vi "Sandbox.vi"() -> ()   [LabVIEW 2019, in "Logger.lvclass"]
uses:
  Logger.lvclass
  ObjData.ctl
  ObjType.ctl
  SignalData.ctl
  EventData.ctl
  TypeDef/AlarmType.ctl
  Database_Postgress_class/Database_Postgress.lvclass
  D:/GIT H4000/H4000/src/DatabaseInterface_class/DatabaseInterface.lvclass
  Database_Postgress_class/Connection Info.ctl
  Logger.lvclass/Logger.ctl
  DatabaseInterface_class/DatabaseInterface.lvclass
panel:
  in  "Events 2":T1[](array[typedef])=[{"obj_tag"="o_tag_1", "event_tag"="o_tag_1_di", "Description"="dsfsadf", "ALARM TYPE"=enum."Alarm", "Value DBL"=234.0, "Value INT"=23423, "Value STR"="xfddf", "Time Stamp"=timestamp(3831350232.4442434 s since 1904-01-01)}]
  in  "sig":T3[](array[typedef])=[{"Value"=1.0, "SignalTag"="s_tag_1", "ObjTag"="o_tag_1", "Desc"="dfs", "Time Stamp"=timestamp(3831177088.422016 s since 1904-01-01)}, {"Value"=2.0, "SignalTag"="s_tag_1", "ObjTag"="o_tag_1", "Desc"="dfas", "Time Stamp"=timestamp(3831263490.641324 s since 1904-01-01)}, {"Value"=3.0, "SignalTag"="s_tag_2", "ObjTag"="o_tag_1", "Desc"="dfsd", "Time Stamp"=timestamp(3830140293.1623626 s since 1904-01-01)}]
  in  "Array":T4[](array[typedef])=[{"object_tag"="o_tag", "parent_tag"="p_tag", "object_type"=enum."Device", "description"="Тестовый обект"}]
  out "error out":errorcluster
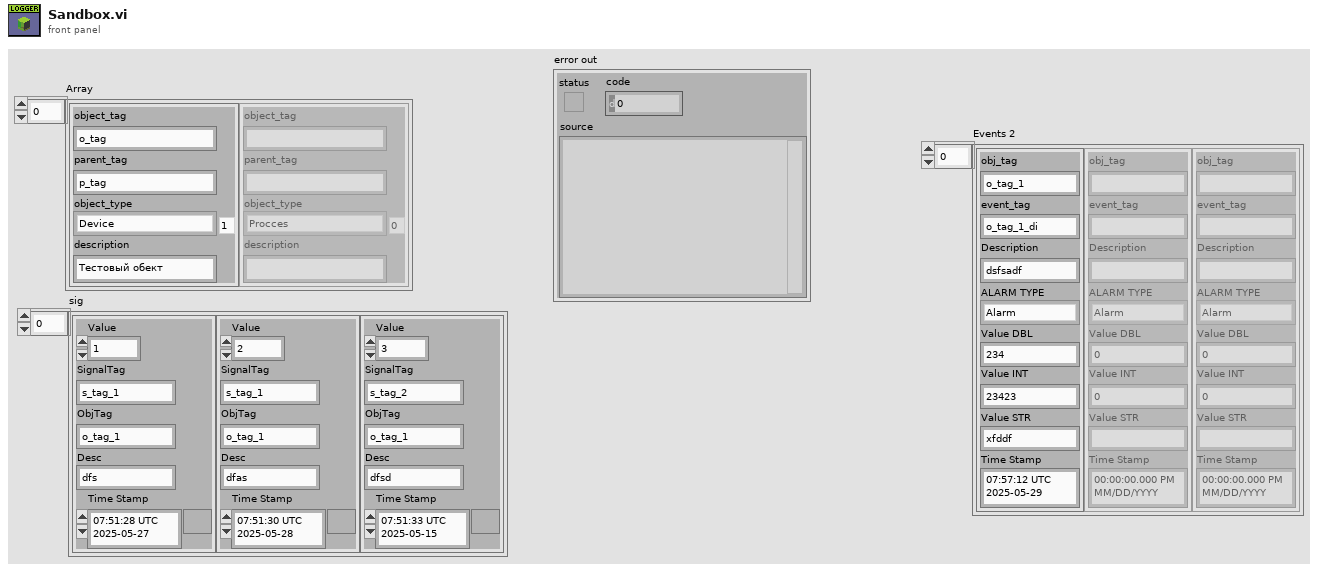
[diagram p1: front panel]
types:
  T1 = typedef "Logger.lvclass/EventData.ctl" = cluster{"obj_tag":string, "event_tag":string, "Description":string, "ALARM TYPE":T2, "Value DBL":dbl, "Value INT":i32, "Value STR":string, "Time Stamp":timestamp}
  T2 = typedef "AlarmType.ctl" = enum16{"Normal", "Warning", "Alarm"}
  T3 = typedef "Logger.lvclass/SignalData.ctl" = cluster{"Value":dbl, "SignalTag":string, "ObjTag":string, "Desc":string, "Time Stamp":timestamp}
  T4 = typedef "Logger.lvclass/ObjData.ctl" = cluster{"object_tag":string, "parent_tag":string, "object_type":T5, "description":string}
  T5 = typedef "Logger.lvclass/ObjType.ctl" = enum16{"Procces", "Device", "Signal", "DI", "DO", "DA", "AI", "AO", "AA"}
  T6 = typedef "DatabaseInterface.lvclass/Connection Info.ctl" = cluster{"IP_Address":string, "Port":u16, "Timeout":i32, "User":string, "Password":string, "Database":string}
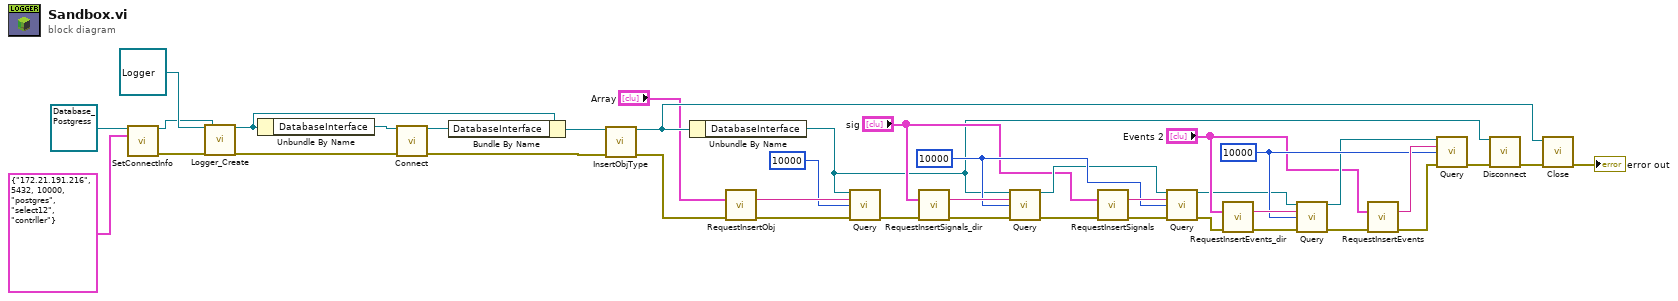
[diagram p0: block diagram]
diagram:
  w8 = 10000 ("Timeout")
  w18 = 10000 ("Timeout")
  n1 = call-dynamic "SetConnectInfo.vi"("reference in"=refnum<class "Database_Postgress.lvclass"> refnum, "Connection Info"=T6 {"IP_Address"="172.21.191.216", "Port"=5432, "Timeout"=10000, "User"="postgres", "Password"="select12", "Database"="contrller"}) -> ("reference out"=w35:refnum<class "Database_Postgress.lvclass">, "error out"=w37:errorcluster)  [unwired: 12 in]
  n2 = call "Logger_Create.vi"("reference in"=refnum<class "Logger.lvclass"> refnum, "error in (no error)"=w37, "DatabaseInterface"=w35) -> ("reference out"=w31:refnum<class "Logger.lvclass">, "error out"=w33:errorcluster)  [unwired: 15 in]
  n3 = Unbundle By Name(w31) -> ("DatabaseInterface"=w34:refnum<class "DatabaseInterface.lvclass">)
  n4 = call-dynamic "Connect.vi"("reference in"=w34, "error in (no error)"=w33) -> ("reference out"=w28:refnum<class "DatabaseInterface.lvclass">, "error out"=w30:errorcluster)  [unwired: 12 in]
  n5 = Bundle By Name(cluster=w31, "DatabaseInterface"=w28) -> (w29:refnum<class "Logger.lvclass">)
  n6 = call "InsertObjType.vi"("reference in"=w29, "error in (no error)"=w30) -> ("reference out"=w27:refnum<class "Logger.lvclass">, "error out"=w22:errorcluster)  [unwired: 11 in, 1 out]
  n7 = Unbundle By Name(w27) -> ("DatabaseInterface"=w13:refnum<class "DatabaseInterface.lvclass">)
  n8 = call "RequestInsertObj.vi"("Array"="Array", "error in (no error)"=w22) -> ("request"=w25:string, "error out"=w26:errorcluster)  [unwired: 12 in]
  n9 = call-dynamic "Query.vi"("reference in"=w13, "Query"=w25, "Timeout"=10000, "error in (no error)"=w26) -> ("error out"=w12:errorcluster)  [unwired: 9 in, 2 out]
  n10 = call "RequestInsertSignals_dir.vi"("Signals"="sig", "error in (no error)"=w12) -> ("request"=w19:string, "error out"=w16:errorcluster)  [unwired: 12 in]
  n11 = call-dynamic "Query.vi"("reference in"=w13, "Query"=w19, "Timeout"=w18, "error in (no error)"=w16) -> ("reference out"=w17:refnum<class "DatabaseInterface.lvclass">, "error out"=w15:errorcluster)  [unwired: 9 in, 1 out]
  n12 = call "RequestInsertSignals.vi"("Events"="sig", "error in (no error)"=w15) -> ("request"=w20:string, "error out"=w21:errorcluster)  [unwired: 12 in]
  n13 = call-dynamic "Query.vi"("reference in"=w17, "Query"=w20, "Timeout"=w18, "error in (no error)"=w21) -> ("reference out"=w3:refnum<class "DatabaseInterface.lvclass">, "error out"=w2:errorcluster)  [unwired: 9 in, 1 out]
  n14 = call "RequestInsertEvents_dir.vi"("Events"="Events 2", "error in (no error)"=w2) -> ("request"=w9:string, "error out"=w6:errorcluster)  [unwired: 12 in]
  n15 = call-dynamic "Query.vi"("reference in"=w3, "Query"=w9, "Timeout"=w8, "error in (no error)"=w6) -> ("reference out"=w7:refnum<class "DatabaseInterface.lvclass">, "error out"=w5:errorcluster)  [unwired: 9 in, 1 out]
  n16 = call "RequestInsertEvents.vi"("Events"="Events 2", "error in (no error)"=w5) -> ("request"=w10:string, "error out"=w11:errorcluster)  [unwired: 12 in]
  n17 = call-dynamic "Query.vi"("reference in"=w7, "Query"=w10, "Timeout"=w8, "error in (no error)"=w11) -> ("error out"=w1:errorcluster)  [unwired: 9 in, 2 out]
  n18 = call-dynamic "Disconnect.vi"("reference in"=w13, "error in (no error)"=w1) -> ("error out"=w32:errorcluster)  [unwired: 12 in, 1 out]
  n19 = call "Close.vi"("error in (no error)"=w32, "Logger in"=w27) -> ("error out"=→"error out":errorcluster)  [unwired: 8 in, 1 out]
